vi "Connect.vi"(8 "error in (no error)":errorcluster, 11 "IgusMotorDrive in":refnum<class "IgusMotorDrive.lvclass">) -> (0 "error out":errorcluster, 2 "Is Connected":bool, 3 "IgusMotorDrive out":refnum<class "IgusMotorDrive.lvclass">)   [LabVIEW 2016, in "IgusMotorDrive.lvclass"]
doc: "This VI establishes a connection to the motor drive.\n\n<b>Copyright (C) 2018 Control Software Solutions Limited. All rights reserved. </b>"
uses:
  IgusMotorDrive.lvclass
  C:/Users/illogicdev/Desktop/IGUS/20190906-1xdryveD1+LABview+ModbusTCP(Gateway)/IgusPositioningSystem Folder/Modules/Classes/motor-drive/MotorDrive.lvclass
  IgusMotorDrive.lvclass/IgusMotorDrive.ctl
  Libraries/Modbus-Master/MB_Master_TCP/MB_Master_TCP.lvclass
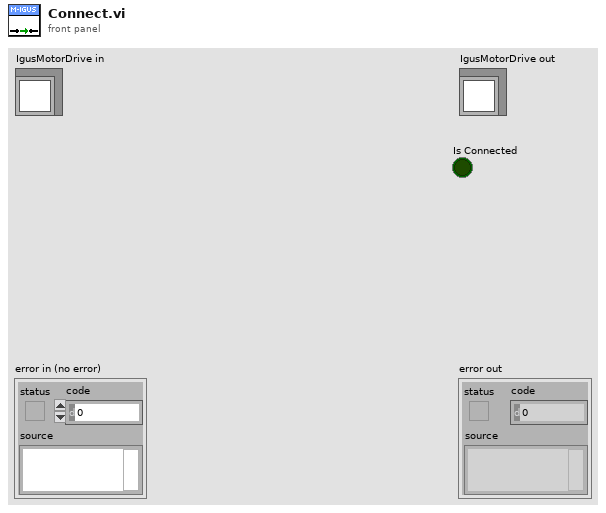
[diagram p1: front panel]
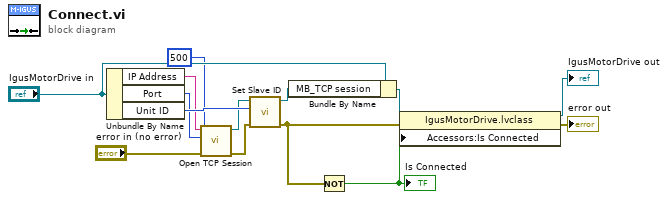
[diagram p0: block diagram]
diagram:
  n1 = Unbundle By Name("IgusMotorDrive in") -> ("IP Address"=w4:string, "Port"=w3:u16, "Unit ID"=w9:u8)
  n2 = call "Open TCP Session.vi"("error in (no error)"="error in (no error)", "Timeout (10000)"=500, "Port (502)"=w3, "IP Address"=w4) -> ("error out"=w5:errorcluster, "MB_TCP session"=w8:refnum<class "MB_Master_TCP.lvclass">)  [unwired: 6 in]
  n3 = call-dynamic "Set Slave ID.vi"("error in (no error)"=w5, "Slave ID"=w9, "MB_TCP_Master in"=w8) -> ("error out"=w6:errorcluster, "MB_TCP_Master out"=w7:refnum<class "MB_Master_TCP.lvclass">)  [unwired: 7 in]
  n4 = Bundle By Name(cluster="IgusMotorDrive in", "MB_TCP session"=w7) -> (w14:refnum<class "IgusMotorDrive.lvclass">)
  n5 = Not(x=w6) -> (.not. x?=w10:bool)
  "Is Connected" <- w10
  n6 = property class="IgusMotorDrive.lvclass"(reference=w14, error in=w6, "Accessors:Is Connected"=w10) -> (reference out=→"IgusMotorDrive out":refnum<class "IgusMotorDrive.lvclass">, error out=→"error out":errorcluster)
